vi "SubVI_SetAtmosphereCorrection.vi"(9 "u8AtmosCorrEnable":u8, 11 "ErrorIn":errorcluster) -> (3 "ErrorOut":errorcluster, 4 "u8Error":u8)   [LabVIEW 2013]
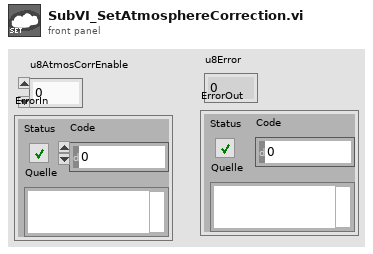
[diagram p1: front panel]
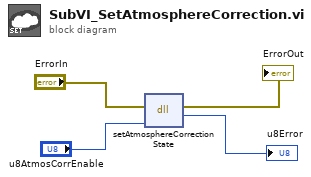
[diagram p0: block diagram]
diagram:
  n1 = dll-call lib="PTH1abs CUsers1000len-bimDesktop&Lieferung_LabView_Interface_11.11.2015Einrichten fÃ¼r - EndkundenDatenTesto_v2013VIlabview_cwrapper_1_0_0.dll" fn="setAtmosphereCorrectionState"(error in="ErrorIn", "u8AtmosCorrEnable"="u8AtmosCorrEnable") -> (error out=→"ErrorOut":errorcluster, "u8Error"=→"u8Error":u8)  [unwired: 3 in, 1 out]
